vi "licz_piq.vi"(8 "b":dbl, 9 "a":dbl, 10 "delta":dbl) -> (1 "Postać kanoniczna":string, 2 "q":dbl, 3 "p":dbl)   [LabVIEW 2020]
doc: "obliczanie p i q"
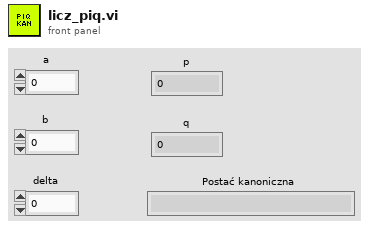
[diagram p1: front panel]
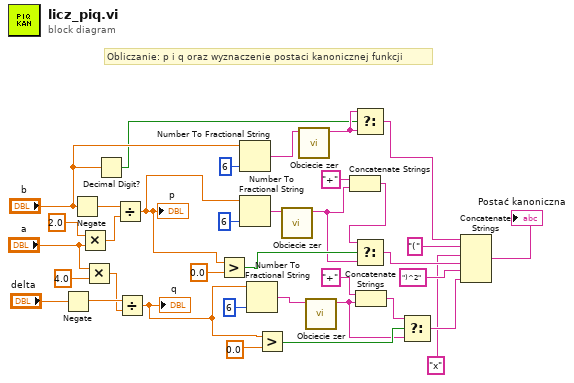
[diagram p0: block diagram]
diagram:
  # "Obliczanie: p i q oraz wyznaczenie postaci kanonicznej funkcji"
  n1 = Negate(x="delta") -> (-x=w32:dbl)
  n2 = Negate(x="b") -> (-x=w36:dbl)
  n3 = Multiply(x=2.0, y="a") -> (x*y=w35:dbl)
  n4 = Multiply(x="a", y=4.0) -> (x*y=w31:dbl)
  n5 = Decimal Digit?(1:"b") -> (0:w5:bool)
  n6 = Divide(x=w36, y=w35) -> (x/y=w3:dbl)
  "p" <- w3
  n7 = Divide(x=w32, y=w31) -> (x/y=w2:dbl)
  "q" <- w2
  n8 = Greater?(x=w3, y=0.0) -> (0:w16:bool)
  n9 = Number To Fractional String(number="b", precision (6)=i16 6) -> (F-format string=w13:string)  [unwired: 2 in]
  n10 = Number To Fractional String(number=w3, precision (6)=i16 6) -> (F-format string=w11:string)  [unwired: 2 in]
  n11 = Number To Fractional String(number=w2, precision (6)=i16 6) -> (F-format string=w9:string)  [unwired: 2 in]
  n12 = Greater?(x=w2, y=0.0) -> (0:w17:bool)
  n13 = call "Obciecie zer.vi"("Wejściowa liczba"=w11) -> ("Wyjściowa liczba"=w10:string)  [unwired: 10 in]
  n14 = call "Obciecie zer.vi"("Wejściowa liczba"=w13) -> ("Wyjściowa liczba"=w12:string)  [unwired: 10 in]
  n15 = call "Obciecie zer.vi"("Wejściowa liczba"=w9) -> ("Wyjściowa liczba"=w8:string)  [unwired: 10 in]
  n16 = Concatenate Strings("+" ("string"), w10) -> (w25:string)
  n17 = Select(t=w12, s=w5, f=w12) -> (s? t:f=w15:string)
  n18 = Select(t=w25, s=w16, f=w10) -> (s? t:f=w24:string)
  n19 = Concatenate Strings("+" ("string"), w8) -> (w20:string)
  n20 = Select(t=w20, s=w17, f=w8) -> (s? t:f=w19:string)
  n21 = Concatenate Strings(w15, "(" ("string"), "x" ("string"), w24, ")^2" ("string"), w19) -> (→"Postać kanoniczna":string)
